vi "Write EventFilter Reference.vi"(10 "EventFilter Reference":T1, 11 "IEventHandler in":refnum<class "IEventHandler.lvclass">) -> (3 "IEventHandler out":refnum<class "IEventHandler.lvclass">)   [LabVIEW 2020, in "ActorEvents.lvlib" / "IEventHandler.lvclass"]
uses:
  <vilib>/gpm_packages/@cs/mva-viewable/Source/ActorEvents/IEventHandler/IEventHandler.lvclass
  <vilib>/gpm_packages/@cs/mva-viewable/Source/ActorEvents/IEventFilter/EventFilter Reference.ctl
  <vilib>/gpm_packages/@cs/mva-viewable/Source/ActorEvents/IEventFilter/IEventFilter.lvclass
  <vilib>/gpm_packages/@cs/mva-viewable/Source/ActorEvents/IEventHandler/IEventHandler.lvclass/IEventHandler.ctl
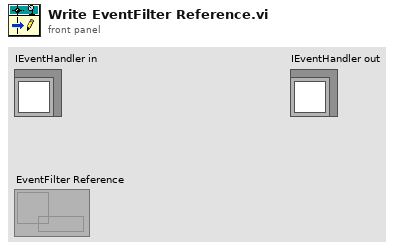
[diagram p1: front panel]
types:
  T1 = typedef "ActorEvents.lvlib/IEventFilter.lvclass/EventFilter Reference.ctl" = refnum<data-value>
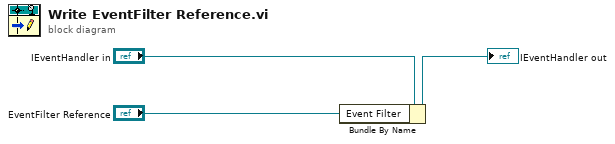
[diagram p0: block diagram]
diagram:
  n1 = Bundle By Name(cluster="IEventHandler in", "Event Filter"="EventFilter Reference") -> (→"IEventHandler out":refnum<class "IEventHandler.lvclass">)
